vi "FakeUnit.vi"(10 "Input":string) -> (2 "Output":string)   [LabVIEW 2019, in "CodeCoverageTestSupport.lvlib"]
uses:
  CodeCoverageTestSupport.lvlib
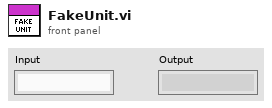
[diagram p1: front panel]
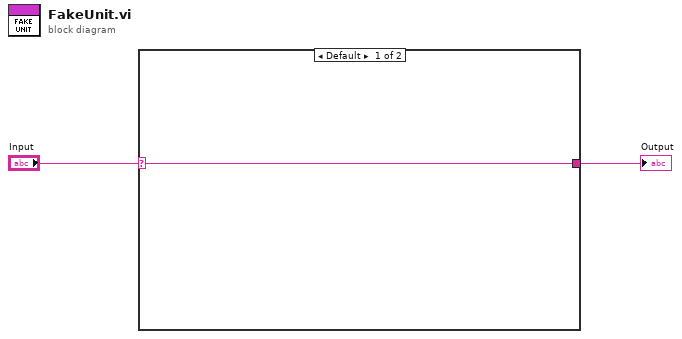
[diagram p0: block diagram]
diagram:
  n1 = case shown="Default" "Input" {
    selector: "Input" -> [w3 w4]
    tunnel: [w3 w4] -> w1
    frame Default {
    }
    frame "True" {
    }
  }
  "Output" <- w1
